vi "Basic 7.vi"() -> ()   [LabVIEW 2014, in "Arduino TFT.lvlib"]
uses:
  <vilib>/Aledyne-TSXperts/Arduino Compatible Compiler for LabVIEW/addons/Arduino TFT/Arduino TFT.lvlib
panel:
  out "Error Out":errorcluster
  in  "Error In":errorcluster
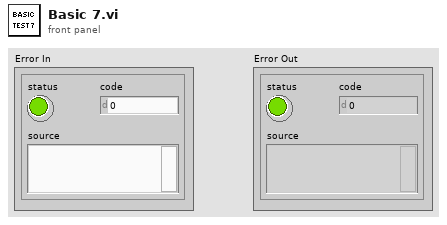
[diagram p1: front panel]
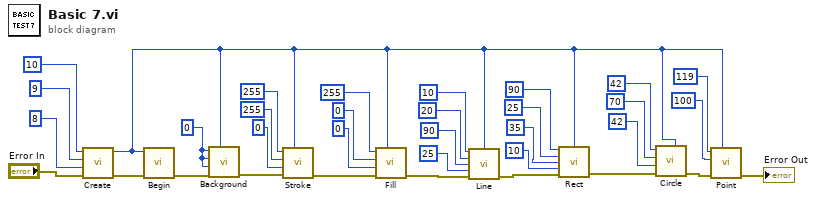
[diagram p0: block diagram]
diagram:
  w2 = u8 0 ("red")
  n1 = call <vilib>:"Create.vi"("Error In"="Error In", "rst"=u8 8 ("cs"), "rs"=u8 9 ("cs"), "cs"=u8 10) -> ("Error Out"=w30:errorcluster, "Instance"=w1:u32)  [unwired: 4 in]
  n2 = call <vilib>:"Begin.vi"("Error In"=w30, "Instance"=w1) -> ("Error Out"=w4:errorcluster)  [unwired: 8 in]
  n3 = call <vilib>:"Background.vi"("Instance"=w1, "Error In"=w4, "blue"=w2, "green"=w2, "red"=w2) -> ("Error Out"=w3:errorcluster)  [unwired: 6 in]
  n4 = call <vilib>:"Stroke.vi"("Instance"=w1, "Error In"=w3, "blue"=u8 0 ("red"), "green"=u8 255 ("red"), "red"=u8 255) -> ("Error Out"=w29:errorcluster)  [unwired: 6 in]
  n5 = call <vilib>:"Fill.vi"("Instance"=w1, "Error In"=w29, "blue"=u8 0 ("red"), "green"=u8 0 ("red"), "red"=u8 255) -> ("Error Out"=w28:errorcluster)  [unwired: 6 in]
  n6 = call <vilib>:"Line.vi"("xStart"=i16 10, "Instance"=w1, "yStart"=i16 20 ("xStart"), "xEnd"=i16 90 ("xStart"), "yEnd"=i16 25 ("xStart"), "Error In"=w28) -> ("Error Out"=w27:errorcluster)  [unwired: 9 in]
  n7 = call <vilib>:"Rect.vi"("x"=i16 90 ("xStart"), "Instance"=w1, "y"=i16 25 ("xStart"), "width"=i16 35 ("xStart"), "height"=i16 10 ("xStart"), "Error In"=w27) -> ("Error Out"=w26:errorcluster)  [unwired: 9 in]
  n8 = call <vilib>:"Circle.vi"("Instance"=w1, "Error In"=w26, "r"=i16 42 ("xStart"), "y"=i16 70 ("xStart"), "x"=i16 42 ("xStart")) -> ("Error Out"=w25:errorcluster)  [unwired: 6 in]
  n9 = call <vilib>:"Point.vi"("Instance"=w1, "Error In"=w25, "y"=u8 100 ("x"), "x"=u8 119) -> ("Error Out"=→"Error Out":errorcluster)  [unwired: 7 in]
